vi "UV-VIS GetPreAmpGainSD.vi"(4 "error in (no error)":errorcluster, 6 "index":i32, 7 "Control in":refnum<class "CCD_camera.lvclass">) -> (0 "error out":errorcluster, 1 "DLL error code":u32, 2 "gain":sgl format="%.2f", 3 "Control out":refnum<class "CCD_camera.lvclass">)   [LabVIEW 2018, in "CCD_camera.lvclass"]
doc: "For those systems that provide a number of pre amp gains to apply to the data as it is read out; this function retrieves the amount of gain that will be applied if the gain specified by index is selected. The number of gains available can be obtained by calling the <B>GetNumberPreAmpGains</B> function and a specific Gain can be selected using the function <B>SetPreAmpGain</B>.\n\n<B>Parameters:</B>\nindex - gain required\n Valid values: 0 to <B>GetNumberPreAmpGains</B>-1\ngain - gain factor for this index.\n\n<B>Error codes:</B>\nDRV_SUCCESS - Gain returned.\nDRV_NOT_INITIALIZED - System not initialized.\nDRV_ACQUIRING - Acquisition in progress.\nDRV_P1INVALID - Invalid index."
uses:
  CCD_camera.lvclass
  C:/Users/Sergey Denisov/Documents/REPS/TRANCON/Classes/Detector/Detector.lvclass
  Detector.lvclass/Detector.ctl
  Detector.lvclass
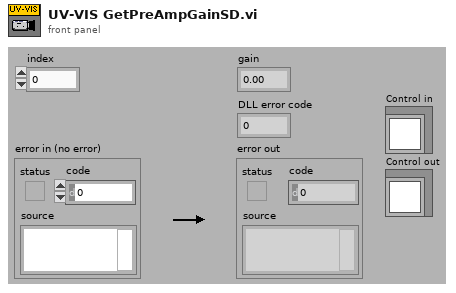
[diagram p1: front panel]
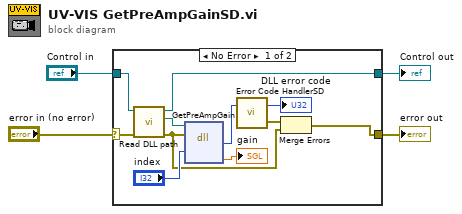
[diagram p0: block diagram]
diagram:
  n1 = case shown="No Error" "error in (no error)" {
    selector: "error in (no error)" -> [w11 w17]
    tunnel: [w7 w17] -> w3
    tunnel: [w5 w16] -> w2
    tunnel: "Control in" -> [w6 w16]
    frame No Error {
      n2 = call "Read DLL path.vi"("error in (no error)"=w11, "Detector in"=w6) -> ("error out"=w8:errorcluster, "DLL path"=w10:path, "Detector out"=w5:refnum<class "CCD_camera.lvclass">)  [unwired: 7 in]
      n3 = dll-call lib="S:/TRANCON/DLL/Atmcd32d.dll" fn="GetPreAmpGain"(path in=w10, error in=w8, "index"="index") -> ("return type"=w15:u32, "gain"=→"gain":sgl)  [unwired: 3 in, 2 out]
      n4 = call "Error Code HandlerSD.vi"("DLL error code"=w15) -> ("error out"=w9:errorcluster, "dup DLL error code"=→"DLL error code":u32)  [unwired: 1 in]
      n5 = Merge Errors(w9, w8) -> (w7:errorcluster)
    }
    frame Error {
    }
  }
  "error out" <- w3
  "Control out" <- w2
